vi "ToteTracking.vi"(8 "ColorImage":T2, 9 "GrayScaleImage":T2, 11 "CameraDevRef":T1={"Camera Address"="192.168.0.90", "CameraStatus"={"status"=FALSE, "code"=0, "source"=""}}) -> (2 "LeftMotor":dbl, 3 "RightMotor":dbl)   [LabVIEW 2014]
uses:
  Camera Types.ctl
  <vilib>/vision/Image Controls.llb/IMAQ Image.ctl
  <vilib>/Rock Robotics/WPI/Camera/WPI_CameraDevRef.ctl
  <vilib>/vision/NI_Vision_Development_Module.lvlib
panel:
  out "Original Image":T2(plugin-control)
  out "Masked":T2(plugin-control)
  in  "Tote Color":T3={"Hue"={23.67058792990901, 48.923317529462665}, "Sat"={66.78571428571429, 255.0}, "Val"={48.571428571428584, 255.0}} {"Hue" scale=0.0..255.0 scale format="%#_3g"}
  out "Particles":i32
  out "Sorted Scores":T4(array[cluster]) {"Carpet" format="%#_3g"; "S" format="%#_3g"; "Trapezoid %" format="%#_3g"; "L" format="%#_3g"; "Area to CH" format="%#_3g"; "X" format="%#_3g"; "Y" format="%#_3g"}
  in  "Annotate":bool=TRUE
  in  "Carpet Color":T5(tab)
  in  "Red":T3={"Hue"={231.0, 14.0}, "Sat"={83.0, 255.0}, "Val"={52.5, 255.0}} {"Hue" scale=0.0..255.0 scale format="%#_3g"}
  in  "Blue":T3={"Hue"={119.0, 181.0}, "Sat"={33.0, 255.0}, "Val"={48.571428571428584, 255.0}} {"Hue" scale=0.0..255.0 scale format="%#_3g"}
  in  "Show Carpet Mask":bool=TRUE
  in  "Score Threshold":dbl=75.0
  out "Detected Totes":T6(array[cluster]) {"Normalized Rect"."Numeric 5" format="%#_2g"; "Normalized Rect"."Numeric 3" format="%#_2g"; "Normalized Rect"."Numeric 2" format="%#_2g"; "Normalized Rect"."Numeric" format="%#_2g"}
  in  "Aspect Fudge Factor":dbl=1.0
  in  "Camera Type":T7=enum."MS HD3000 square"
  in  "Limit Tests?":bool=TRUE
  # "Aspect Ratio"
  # "Density Profile"
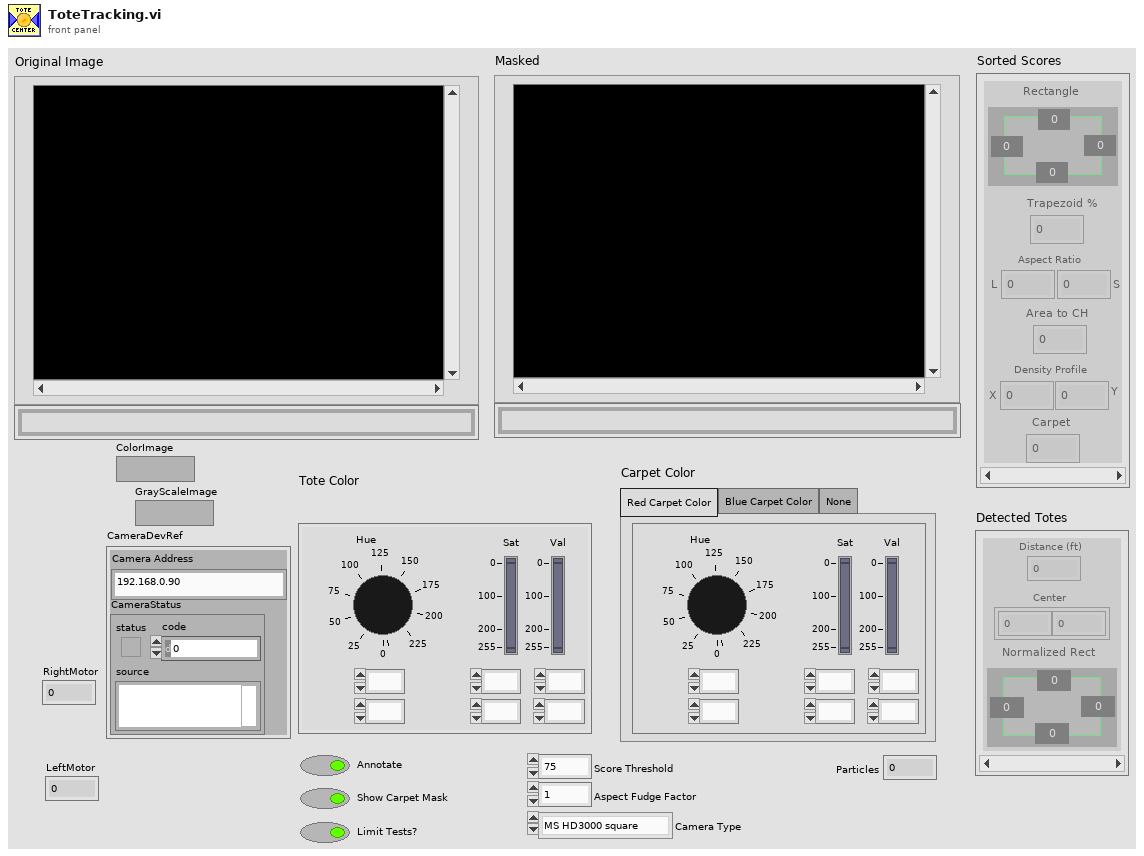
[diagram p1: front panel]
types:
  T1 = typedef "WPI_CameraDevRef.ctl" = cluster{"Camera Address":string, "CameraStatus":errorcluster}
  T2 = typedef "IMAQ Image.ctl" = refnum<image>
  T3 = cluster{"Hue":cluster{dbl, dbl}, "Sat":cluster{dbl, dbl}, "Val":cluster{dbl, dbl}}
  T4 = cluster{"Rectangle":cluster{"Numeric":dbl, "Numeric 2":dbl, "Numeric 3":dbl, "Numeric 5":dbl}, "Trapezoid %":dbl, "L":dbl, "S":dbl, "Area to CH":dbl, "X":dbl, "Y":dbl, "Carpet":dbl}[]
  T5 = enum32{"Red Carpet Color", "Blue Carpet Color", "None"}
  T6 = cluster{"Distance (ft)":dbl, "Center":cluster{dbl, dbl}, "Normalized Rect":cluster{"Numeric":dbl, "Numeric 2":dbl, "Numeric 3":dbl, "Numeric 5":dbl}}[]
  T7 = typedef "Camera Types.ctl" = enum16{"206", "1011", "1013", "MS HD3000 square", "MS HD3000 640x480"}
  T8 = typedef "Particle Parameters" = i32
  T9 = typedef "Image Type" = u32
  T10 = cluster{"Bounding box":cluster{"left":dbl, "top":dbl, "right":dbl, "bottom":dbl}, "Trapezoid":dbl, "Long Aspect":dbl, "Short Aspect":dbl, "Area to CH":dbl, "X Mask":dbl, "Y Mask":dbl, "Carpet":dbl}[]
  T11 = cluster{"Red":cluster{"Hue":cluster{dbl, dbl}, "Sat":cluster{dbl, dbl}, "Val":cluster{dbl, dbl}}, "Blue":cluster{"Hue":cluster{dbl, dbl}, "Sat":cluster{dbl, dbl}, "Val":cluster{dbl, dbl}}}
  T12 = cluster{cluster{"[0]":dbl, "[1]":dbl, "[2]":dbl, "[3]":dbl}, "Score":dbl, "Long Edge Score":dbl, "Short Edge Score":dbl, dbl, "X Score":dbl, "Y Score":dbl, "Carpet":dbl}[]
  T13 = cluster{"Distance (ft)":dbl, "Center":cluster{"X":dbl, "Y":dbl}, "Normalized Rect":cluster{"Numeric":dbl, "Numeric 2":dbl, "Numeric 3":dbl, "Numeric 5":dbl}}[]
  T14 = cluster{"Distance (ft)":dbl, "Center":cluster{"X":dbl, "Y":dbl}, "Normalized Rect":cluster{"Numeric":dbl, "Numeric 2":dbl, "Numeric 3":dbl, "Numeric 5":dbl}}
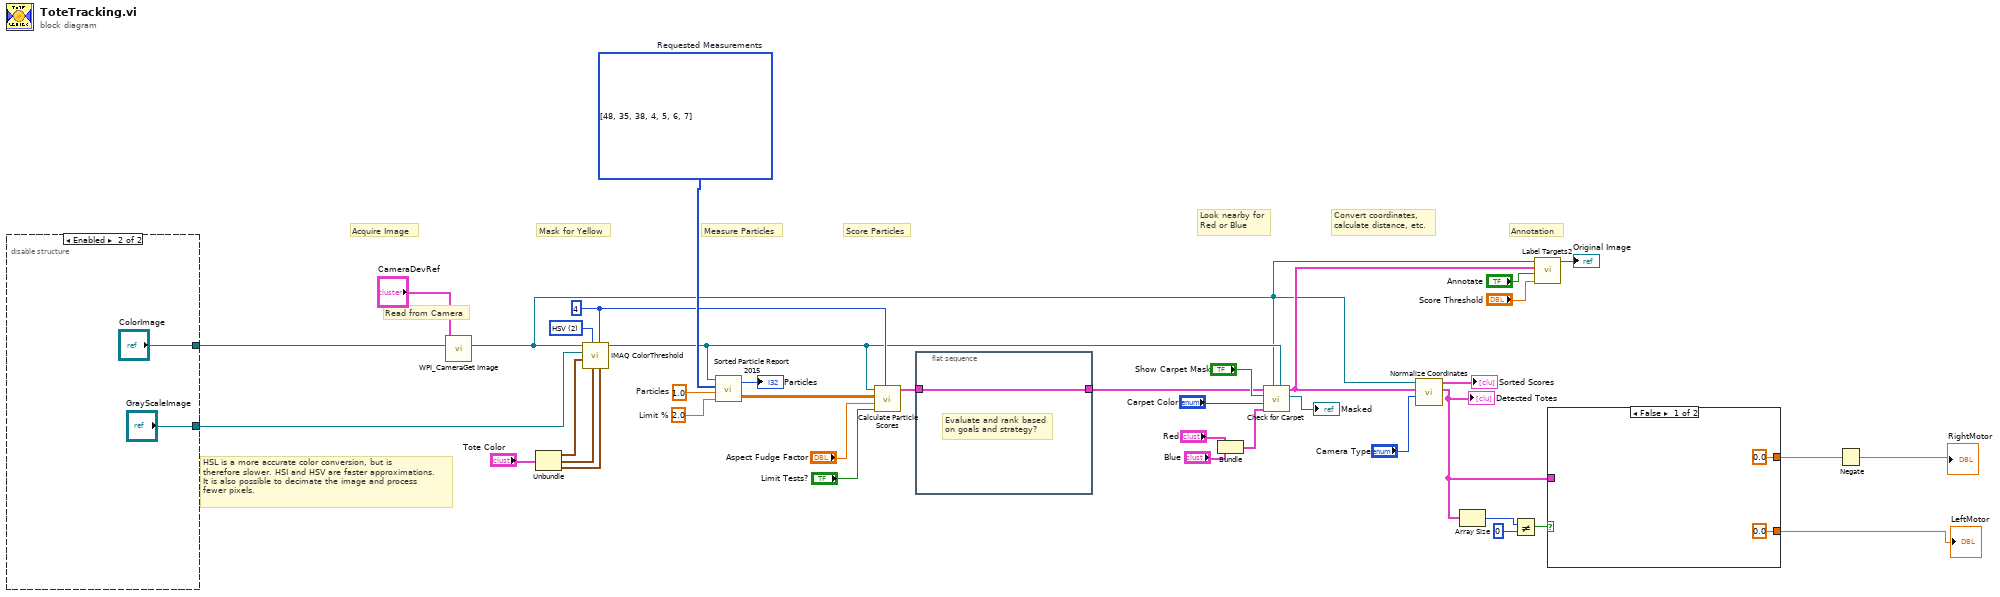
[diagram p0: block diagram]
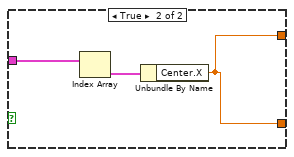
[diagram p2: hidden frame]
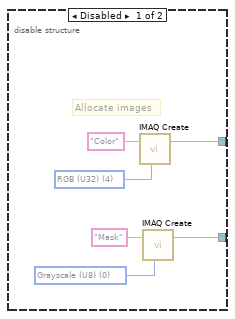
[diagram p3: hidden frame]
diagram:
  w19 = 4 ("Replace Value")
  w28 = 2.0  # Limit %
  w31 = 1.0  # Particles
  w36 = u16 2 items=["RGB", "HSL", "HSV", "HSI"] ("Color Mode")
  w37 = T8[] [48, 35, 38, 4, 5, 6, 7] items=["Center of Mass X", "Center of Mass Y", "First Pixel X", "First Pixel Y", "Bounding Rect Left", "Bounding Rect Top", "Bounding Rect Right", "Bounding Rect Bottom", "Max Feret Diameter Start X", "Max Feret Diameter Start Y", "Max Feret Diameter End X", "Max Feret Diameter End Y", "Max Horiz. Segment Length Left", "Max Horiz. Segment Length Right", "Max Horiz. Segment Length Row", "-", "Bounding Rect Width", "Bounding Rect Height", "Bounding Rect Diagonal", "Perimeter", "Convex Hull Perimeter", "Holes' Perimeter", "Max Feret Diameter", "Equivalent Ellipse Major Axis", "Equivalent Ellipse Minor Axis", "Equivalent Ellipse Minor Axis (Feret)", "Equivalent Rect Long Side", "Equivalent Rect Short Side", "Equivalent Rect Diagonal", "Equivalent Rect Short Side (Feret)", "Average Horiz. Segment Length", "Average Vert. Segment Length", "Hydraulic Radius", "Waddel Disk Diameter", "-", "Area", "Holes' Area", "Particle & Holes' Area", "Convex Hull Area", "Image Area", "-", "Number of Holes", "Number of Horiz. Segments", "Number of Vert. Segments", "-", "Orientation", "Max Feret Diameter Orientation", "-", "% Area/Image Area", "% Area/(Particle & Holes' Area)", "Ratio of Equivalent Ellipse Axes", "Ratio of Equivalent Rect Sides", "-", "Elongation Factor", "Compactness Factor", "Heywood Circularity Factor", "Type Factor", "-", "Sum X", "Sum Y", "Sum XX", "Sum XY", "Sum YY", "Sum XXX", "Sum XXY", "Sum XYY", "Sum YYY", "-", "Moment of Inertia XX", "Moment of Inertia XY", "Moment of Inertia YY", "Moment of Inertia XXX", "Moment of Inertia XXY", "Moment of Inertia XYY", "Moment of Inertia YYY", "Norm. Moment of Inertia XX", "Norm. Moment of Inertia XY", "Norm. Moment of Inertia YY", "Norm. Moment of Inertia XXX", "Norm. Moment of Inertia XXY", "Norm. Moment of Inertia XYY", "Norm. Moment of Inertia YYY", "Hu Moment 1", "Hu Moment 2", "Hu Moment 3", "Hu Moment 4", "Hu Moment 5", "Hu Moment 6", "Hu Moment 7"]  # Requested Measurements
  # "Read from Camera"
  # "Measure Particles"
  # "Convert coordinates,\ncalculate distance, etc."
  # "Annotation"
  # "Score Particles"
  # "Mask for Yellow"
  # "Acquire Image"
  # "HSL is a more accurate color conversion, but is\ntherefore slower. HSI and HSV are faster approximations.\nIt is also possible to decimate the image and process\nfewer pixels."
  # "Look nearby for\nRed or Blue"
  n1 = disable-structure shown="Enabled" {
    disable-tunnel: [w43 "ColorImage"] -> w39
    disable-tunnel: [w40 "GrayScaleImage"] -> w38
    frame Disabled {
      w42 = T9 0 items=["Grayscale (U8)", "Grayscale (I16)", "Grayscale (SGL)", "Complex (CSG)", "RGB (U32)", "HSL (U32)", "RGB (U64)", "Grayscale (U16)"] ("Image Type")
      w44 = T9 4 items=["Grayscale (U8)", "Grayscale (I16)", "Grayscale (SGL)", "Complex (CSG)", "RGB (U32)", "HSL (U32)", "RGB (U64)", "Grayscale (U16)"] ("Image Type")
      # "Allocate images"
      n2 = call "IMAQ Create"("Image Name"="Color", "Image Type"=w44) -> ("New Image"=w43:T2)  [unwired: 2 in, 2 out]
      n3 = call "IMAQ Create"("Image Name"="Mask", "Image Type"=w42) -> ("New Image"=w40:T2)  [unwired: 2 in, 2 out]
    }
    frame Enabled {
    }
  }
  n4 = call <vilib>:"WPI_CameraGet Image.vi"("Image"=w39, "CameraDevRef"="CameraDevRef") -> ("Image Out"=w11:T2)  [unwired: 7 in, 2 out]
  n5 = Unbundle("Tote Color") -> ("Hue"=w35:cluster{dbl, dbl}, "Sat"=w34:cluster{dbl, dbl}, "Val"=w33:cluster{dbl, dbl})
  n6 = call "IMAQ ColorThreshold"("Blue or Luma or Val or Inten Range"=w33, "Replace Value"=w19, "Green or Sat Range"=w34, "Color Mode"=w36, "Red or Hue Range"=w35, "Image Dst"=w38, "Image Src"=w11) -> ("Image Dst Out"=w12:T2)  [unwired: 3 in, 1 out]
  n7 = call "Sorted Particle Report 2015.vi"("Min Area Size %"=w28, "Particle Count Limit"=w31, "Pixel Measurements"=w37, "Image in"=w12) -> ("Sorted Data"=w29:dbl[][], "Particles"=→"Particles":i32)
  n8 = call "Calculate Particle Scores.vi"("Pixel Value"=w19, "Limit Tests?"="Limit Tests?", "Aspect Fudge Factor"="Aspect Fudge Factor", "Sorted Data"=w29, "Image in"=w12) -> ("Scores"=w14:T10)  [unwired: 6 in]
  n9 = flat-sequence {
    tunnel: w14 -> [w48]
    tunnel: [w48] -> w13
    frame #0 {
      # "Evaluate and rank based\non goals and strategy?"
    }
  }
  n10 = Bundle("Red"="Red", "Blue"="Blue") -> (w20:T11)  [unwired: 1 in]
  n11 = call "Check for Carpet.vi"("Original Mask"=w12, "Original Color"=w11, "Carpet Colors"=w20, "Carpet Selector"="Carpet Color", "Combine Carpet Mask"="Show Carpet Mask", "Initial Scores"=w13) -> ("Updated Mask"=→"Masked":T2, "Updated Scores"=w18:T12)  [unwired: 4 in]
  n12 = call "Normalize Coordinates.vi"("Camera Type"="Camera Type", "Targets"=w18, "Image in"=w11) -> ("Found Totes"=w8:T13, "Sorted Scores"=→"Sorted Scores":T4)  [unwired: 7 in]
  "Detected Totes" <- w8
  n13 = Array Size(array=w8) -> (size(s)=w7:i32)
  n14 = Not Equal?(x=w7, y=0) -> (x != y?=w5:bool)
  n15 = call "Label Targets2.vi"("Score Threshold"="Score Threshold", "Annotate"="Annotate", "Targets"=w18, "Image in"=w11) -> ("Image out"=→"Original Image":T2)  [unwired: 7 in]
  n16 = case shown="False" w5 {
    tunnel: w8 -> [_ w52]
    tunnel: [0.0 ("X") w51] -> w4
    tunnel: [0.0 ("X") w51] -> w3
    frame False {
    }
    frame True {
      n17 = Index Array(array=w52) -> (element=w53:T14)  [unwired: 1 in]
      n18 = Unbundle By Name(w53) -> ("Center.X"=w51:dbl)
    }
  }
  "LeftMotor" <- w3
  n19 = Negate(x=w4) -> (-x=→"RightMotor":dbl)
